vi "Open Fcurve object.vi"(6 "wait for reply (T)":bool=TRUE, 7 "Channel datum out":waveform(dbl)[](array[waveform]), 8 "error in":errorcluster, 9 "Channel name(s)":string[](array[string]), 10 "Group metadata":T2) -> (0 "error out":errorcluster, 1 "timed out?":bool, 2 "Metadata out":T1, 3 "Fcurve out":cluster{"X":dbl[], "Y":dbl[]}[](array[cluster]))   [LabVIEW 2019, in "Analysis.lvlib"]
doc: "_____\nCreated using DQMH Event Scripter 6.1.0.128."
uses:
  Analysis.lvlib
  Class Library/TDMS_DataHandler_class/Fcurve Meta data.ctl
  Class Library/Fcurve_class/Metadata.ctl
  Open Fcurve object Argument--cluster.ctl
  Open Fcurve object (Reply Payload)--cluster.ctl
  Class Library/TDMS_DataHandler_class/TDMS_DataHandler.lvclass
  Class Library/Fcurve_class/Fcurve.lvclass
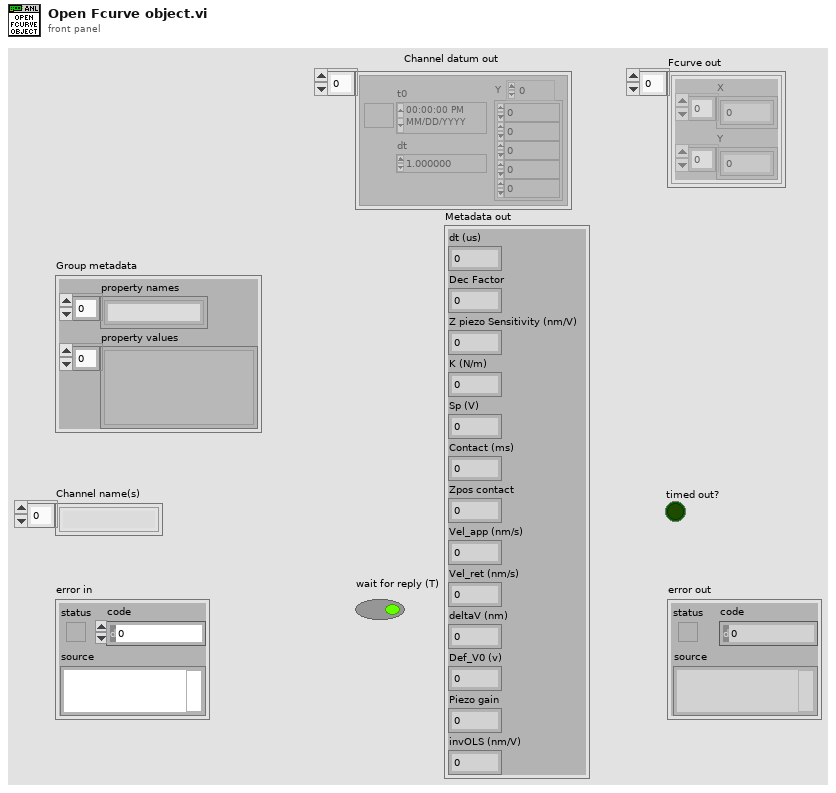
[diagram p1: front panel]
types:
  T1 = typedef "Fcurve.lvclass/Metadata.ctl" = cluster{"dt (us)":dbl, "Dec Factor":dbl, "Z piezo Sensitivity (nm/V)":dbl, "K (N/m)":dbl, "Sp (V)":dbl, "Contact (ms)":dbl, "Zpos contact":dbl, "Vel_app (nm/s)":dbl, "Vel_ret (nm/s)":dbl, "deltaV (nm)":dbl, "Def_V0 (v)":dbl, "Piezo gain":dbl, "invOLS (nm/V)":dbl}
  T2 = typedef "TDMS_DataHandler.lvclass/Fcurve Meta data.ctl" = cluster{"property names":string[], "property values":variant[]}
  T3 = typedef "Analysis.lvlib/Open Fcurve object Argument--cluster.ctl" = cluster{"Group metadata":T2, "Channel name(s)":string[], "Channel datum out":waveform(dbl)[], "Wait Notifier":refnum<notifier>, "wait for reply":bool}
  T4 = typedef "Analysis.lvlib/Request Events--cluster.ctl" = cluster{"Stop Module":refnum<user-event>, "Show Panel":refnum<user-event>, "Hide Panel":refnum<user-event>, "Get Module Execution Status":refnum<user-event>, "Show Diagram":refnum<user-event>, "Wakeup Helper Loop":refnum<user-event>, "Change Settings":refnum<user-event>, "Update analysis parameters":refnum<user-event>, "Update Savitzky parameters":refnum<user-event>, "Update decimation":refnum<user-event>, "Update contact parameters":refnum<user-event>, "Update Tau delay (ms)":refnum<user-event>, "Open Fcurve object":refnum<user-event>, "Apply Savitzky Golay Filter":refnum<user-event>, "Apply decimation":refnum<user-event>}
  T5 = typedef "Analysis.lvlib/Open Fcurve object (Reply Payload)--cluster.ctl" = cluster{"Fcurve out":cluster{"X":dbl[], "Y":dbl[]}[], "Metadata out":T1, "error":errorcluster}
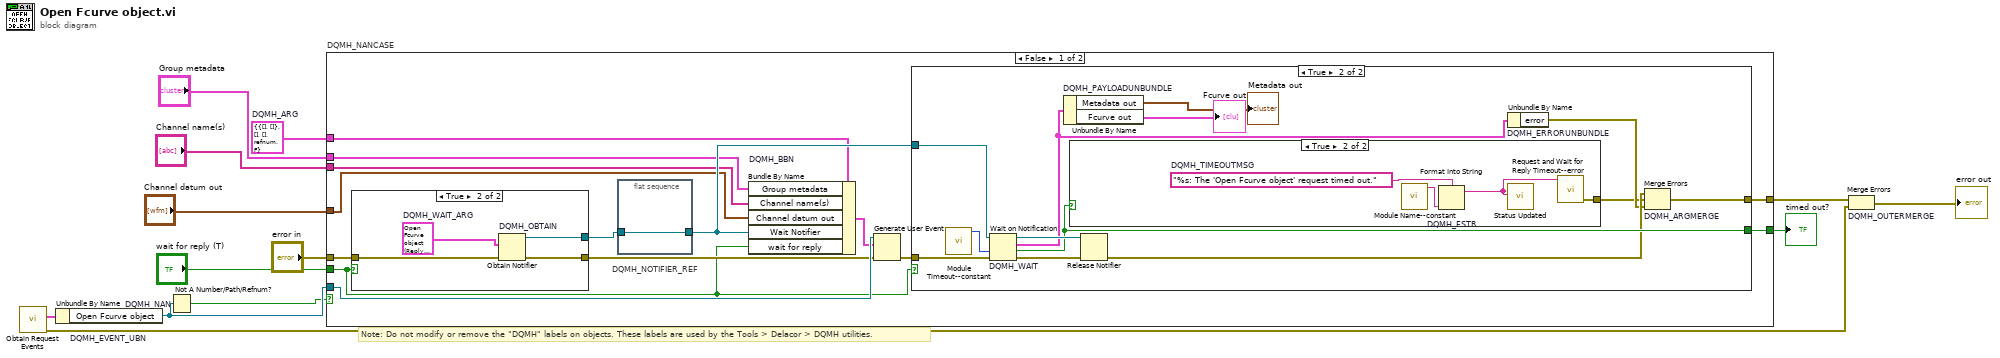
[diagram p0: block diagram]
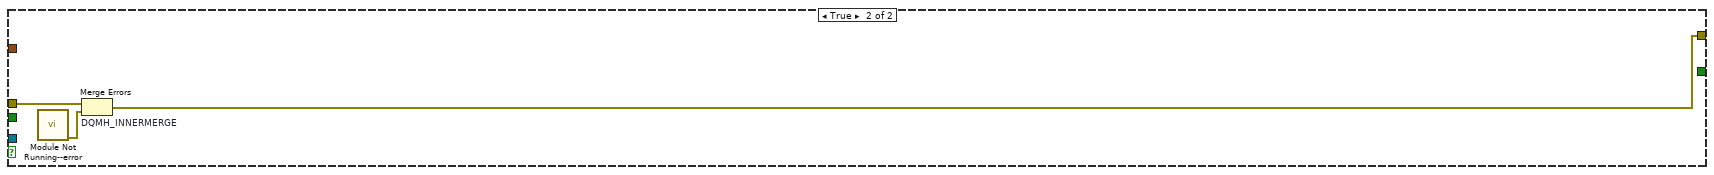
[diagram p5: hidden frame]
diagram:
  w7 = T3 {"Group metadata"={"property names"=[], "property values"=[]}, "Channel name(s)"=[], "Channel datum out"=[], "Wait Notifier"=refnum, "wait for reply"=FALSE}  # DQMH_ARG
  # "Note: Do not modify or remove the \"DQMH\" labels on objects. These labels are used by the Tools > Delacor > DQMH utilities."
  n1 = call "Obtain Request Events.vi"() -> ("error out"=w2:errorcluster, "Analysis Request Events"=w1:T4)  [unwired: 10 in]
  n2 = Unbundle By Name "DQMH_EVENT_UBN"(w1) -> ("Open Fcurve object"=w11:refnum<user-event>)
  n3 = Not A Number/Path/Refnum? "DQMH_NAN"(number/path/refnum=w11) -> (NaN/Path/Refnum?=w10:bool)
  n4 = case "DQMH_NANCASE" shown="False" w10 {
    tunnel: "error in" -> [w27 w54]
    tunnel: w11 -> [w25 _]
    tunnel: [w22 w53] -> w8
    tunnel: [w23 _] -> w9
    tunnel: w7 -> [w18 _]
    tunnel: "Group metadata" -> [w17 _]
    tunnel: "Channel name(s)" -> [w16 _]
    tunnel: "Channel datum out" -> [w15 _]
    tunnel: "wait for reply (T)" -> [w14 _]
    frame False {
      n5 = case shown="True" w14 {
        tunnel: w27 -> [w47 w51]
        tunnel: [w47 w50] -> w24
        tunnel: [_ w48] -> w20
        frame False {
        }
        frame True {
          w49 = T5 {"Fcurve out"=[], "Metadata out"={"dt (us)"=2.0, "Dec Factor"=1.0, "Z piezo Sensitivity (nm/V)"=6000.0, "K (N/m)"=0.6, "Sp (V)"=16.0, "Contact (ms)"=0.0, "Zpos contact"=2.000001, "Vel_app (nm/s)"=10000.0, "Vel_ret (nm/s)"=100000.0, "deltaV (nm)"=600.0, "Def_V0 (v)"=-0.113287, "Piezo gain"=1.0, "invOLS (nm/V)"=23.8}, "error"={"status"=FALSE, "code"=0, "source"=""}}  # DQMH_WAIT_ARG
          n6 = Obtain Notifier "DQMH_OBTAIN"(notification data type=w49, error in (no error)=w51) -> (notifier out=w48:refnum<notifier>, error out=w50:errorcluster)  [unwired: 2 in, 1 out]
        }
      }
      n7 = flat-sequence "DQMH_NOTIFIER_REF" {
        tunnel: w20 -> [w28]
        tunnel: [w28] -> w19
        frame #0 {
        }
      }
      n8 = Bundle By Name "DQMH_BBN"(cluster=w18, "Group metadata"=w17, "Channel name(s)"=w16, "Channel datum out"=w15, "Wait Notifier"=w19, "wait for reply"=w14) -> (w21:T3)
      n9 = Generate User Event(user event=w25, event data cluster=w21, error in=w24) -> (error out=w26:errorcluster)  [unwired: 1 in, 1 out]
      n10 = case shown="True" w14 {
        tunnel: w26 -> [w29 w42]
        tunnel: w19 -> [_ w41]
        tunnel: [_ w39] -> w23
        tunnel: [w29 w38] -> w22
        frame False {
        }
        frame True {
          n11 = call "Module Timeout--constant.vi"() -> ("Module Timeout"=w32:i32)  [unwired: 11 in]
          n12 = Wait on Notification "DQMH_WAIT"(notifier=w41, timeout in ms (-1)=w32, error in (no error)=w42) -> (notifier out=w40:refnum<notifier>, notification=w33:T5, timed out?=w39:bool, error out=w37:errorcluster)  [unwired: 1 in]
          n13 = Unbundle By Name "DQMH_PAYLOADUNBUNDLE"(w33) -> ("Metadata out"=→"Metadata out":T1, "Fcurve out"=→"Fcurve out":cluster{"X":dbl[], "Y":dbl[]}[])
          n14 = case shown="True" w39 {
            tunnel: [_ w44] -> w34
            frame False {
            }
            frame True {
              w46 = "%s: The 'Open Fcurve object' request timed out."  # DQMH_TIMEOUTMSG
              n15 = call "Module Name--constant.vi"() -> ("Module Name"=w43:string)  [unwired: 11 in]
              n16 = Format Into String "DQMH_FSTR"(format string=w46, w43) -> (resulting string=w45:string)  [unwired: 2 in, 1 out]
              n17 = call "Status Updated.vi"("Status"=w45) -> ()  [unwired: 10 in, 1 out]
              n18 = call "Request and Wait for Reply Timeout--error.vi"("Error Message"=w45) -> ("error out"=w44:errorcluster)  [unwired: 10 in]
            }
          }
          n19 = Release Notifier(notifier=w40, error in (no error)=w37) -> (error out=w36:errorcluster)  [unwired: 1 in, 2 out]
          n20 = Unbundle By Name "DQMH_ERRORUNBUNDLE"(w33) -> ("error"=w35:errorcluster)
          n21 = Merge Errors "DQMH_ARGMERGE"(w36, w34, w35) -> (w38:errorcluster)
        }
      }
    }
    frame True {
      n22 = call "Module Not Running--error.vi"() -> ("error out"=w52:errorcluster)  [unwired: 11 in]
      n23 = Merge Errors "DQMH_INNERMERGE"(w54, w52) -> (w53:errorcluster)
    }
  }
  "timed out?" <- w9
  n24 = Merge Errors "DQMH_OUTERMERGE"(w8, w2) -> (→"error out":errorcluster)
